vi "LocalisationExample.vi"() -> ()   [LabVIEW 2013]
panel:
  in  "LocalizedLang":string[](array[string])
  in  "RefWord":string
  in  "LocalizedWord":string
  in  "Ref lang":string[](array[string])
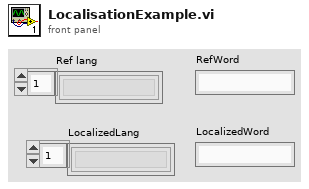
[diagram p1: front panel]
types:
  T1 = cluster{"RefWords":string[], "LocalizedWords":string[]}
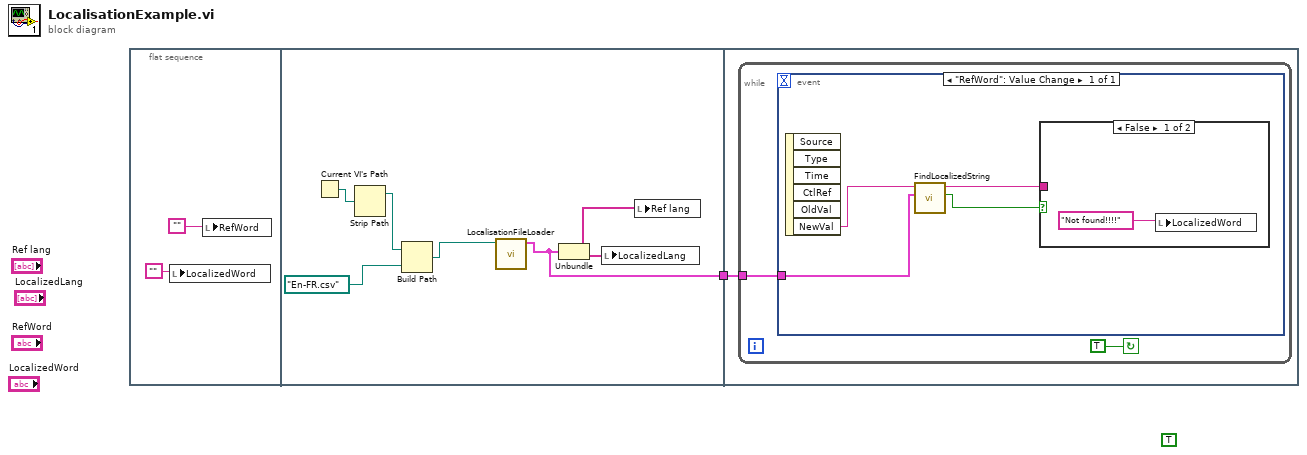
[diagram p0: block diagram]
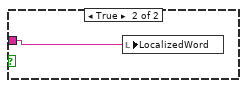
[diagram p2: hidden frame]
diagram:
  (unwired) TRUE
  n1 = flat-sequence {
    tunnel: [w4] -> w1
    tunnel: w1 -> [w11]
    frame #0 {
      n2 = local write "LocalizedWord"("") -> ()
      n3 = local write "RefWord"("") -> ()
    }
    frame #1 {
      n4 = Current VI's Path() -> (path=w10:path)
      n5 = Strip Path(path=w10) -> (stripped path=w9:path)  [unwired: 1 out]
      n6 = Build Path(base path=w9, name or relative path=path "En-FR.csv") -> (appended path=w7:path)
      n7 = call "LocalisationFileLoader.vi"("FilePath"=w7) -> ("LocalisationFileContent[out]"=w4:T1)  [unwired: 9 in, 1 out]
      n8 = Unbundle(w4) -> ("RefWords"=w6:string[], "LocalizedWords"=w5:string[])
      n9 = local write "LocalizedLang"(w5) -> ()
      n10 = local write "Ref lang"(w6) -> ()
    }
    frame #2 {
      n11 = while {
        tunnel: w11 -> [w13]
        stop <- TRUE continue-if-true
        n12 = event shown="[0] \"RefWord\": Value Change" {
          selector: _ -> [_]
          dyn-events: _ -> [_]
          timeout: _ -> [_]
          tunnel: w13 -> [w15]
          event "RefWord": Value Change {
            n13 = event-data() -> ("NewVal"=w16:string)  [unwired: 1 in, 5 out]
            n14 = call "FindLocalizedString.vi"("LocalizationFileContent"=w15, "String[in]"=w16) -> ("Found"=w17:bool, "LocalizedString"=w14:string)  [unwired: 8 in]
            n15 = case shown="False" w17 {
              tunnel: w14 -> [_ w19]
              frame False {
                n16 = local write "LocalizedWord"("Not found!!!!") -> ()
              }
              frame True {
                n17 = local write "LocalizedWord"(w19) -> ()
              }
            }
          }
        }
      }
    }
  }
